vi "About.vi"(10 "FileName (without extension)":string="messagesEN") -> ()   [LabVIEW 2020]
uses:
  Messages/simonMessages/simonMessages.lvclass
  TextDisplay/TextDisplay Class.lvclass
  uiControlsMgr/uiControlsMgr.lvclass
panel:
  out "0009":string caption="MOSTRADOR"
  out "Boolean":bool
  out "Boolean 4":bool
  out "Boolean 3":bool
  out "Boolean 2":bool
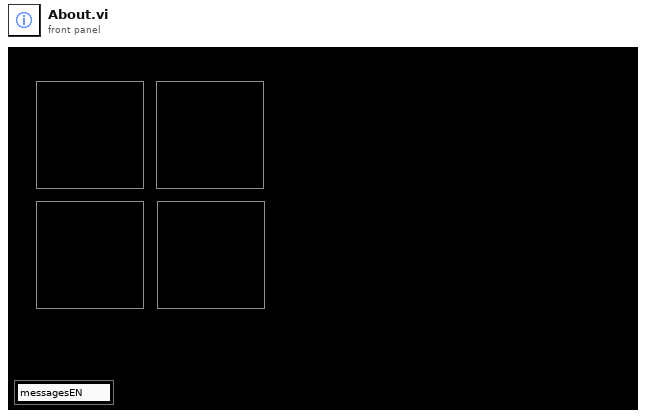
[diagram p1: front panel]
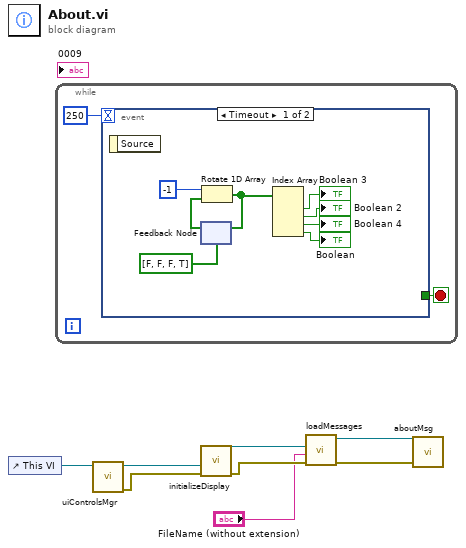
[diagram p0: block diagram]
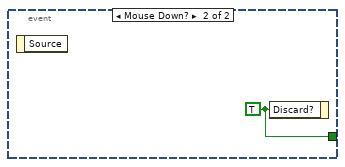
[diagram p2: hidden frame]
diagram:
  n1 = control-ref of="This VI"() -> (w1:refnum<vi>)
  n2 = while {
    stop <- w9 stop-if-true
    n3 = event shown="[0] Timeout" {
      selector: _ -> [_ _]
      dyn-events: _ -> [_ _]
      timeout: 250 -> [_ _]
      tunnel: [_ w19] -> w9
      event Timeout {
        n4 = event-data() -> ()  [unwired: 1 in, 1 out]
        n5 = feedback #1(bool[] [FALSE, FALSE, FALSE, TRUE]) -> (w16:bool[])
        n6 = Rotate 1D Array(1:w16, 2:-1 ("n")) -> (0:w15:bool[])
        n7 = feedback-in #1(w15) -> ()
        n8 = Index Array(array=w15) -> (element #1=→"Boolean 3":bool, element #2=→"Boolean 2":bool, element #3=→"Boolean 4":bool, element #4=→"Boolean":bool)  [unwired: 4 in]
      }
      event Mouse Down? {
        w19 = TRUE ("Discard?")
        n9 = event-data() -> ()  [unwired: 1 in, 1 out]
        n10 = event-data("Discard?"=w19) -> ()  [unwired: 1 in, 1 out]
      }
    }
  }
  n11 = call "uiControlsMgr.vi"("VI reference"=w1) -> ("error out"=w5:errorcluster, "uiControlsMgr out"=w8:refnum<class "uiControlsMgr.lvclass">)  [unwired: 9 in]
  n12 = call "initializeDisplay.vi"("error in (no error)"=w5, "uiControlsMgr.lvclass"=w8) -> ("error out"=w4:errorcluster, "TextDisplay Class out"=w7:refnum<class "TextDisplay Class.lvclass">)  [unwired: 8 in]
  n13 = call "loadMessages.vi"("error in (no error)"=w4, "FileName (without extension)"="FileName (without extension)", "TextDisplay"=w7) -> ("error out"=w6:errorcluster, "simonMessages out"=w2:refnum<class "simonMessages.lvclass">)  [unwired: 7 in]
  n14 = call "aboutMsg.vi"("error in (no error)"=w6, "simonMessages in"=w2) -> ()  [unwired: 8 in, 2 out]
